vi "Training_Baseline_ICA.vi"(0 "Random_Repeat":i32=20, 1 "Random_num":i32=9, 3 "Experimentation_num":i32=2, 4 "rate":dbl=500.0 caption="Rate" format="%0.2f", 5 "Group Number":i32, 6 "Brain_data_source":dbl[](array[numeric]) caption="EEG_Raw_Data" format="%0.3f", 7 "samples per channel":i32=25, 9 "전체_Selected":i32[](array[numeric]), 10 "Selected":i32[](array[numeric]), 11 "Nontarget_Flash_Order":i32[][](array[numeric]), 12 "Target_Flash_Order":i64[](array[numeric]), 13 "W":dbl[][](array[numeric])) -> (14 "Target":dbl[][](array[numeric]), 15 "Nontarget_ERP":dbl[](array[numeric]), 18 "NonTarget":dbl[][](array[numeric]), 19 "Target_ERP":dbl[](array[numeric]))   [LabVIEW 2014]
uses:
  <vilib>/Analysis/3filter.llb/Filter Passband Type.ctl
  <vilib>/Analysis/baseanly.llb/Mean (DBL).vi
  <vilib>/Analysis/3filter.llb/Butterworth Filter (DBL).vi
  <vilib>/Analysis/NI_AALBase.lvlib
  <vilib>/gmath/NI_Gmath.lvlib
  <vilib>/Utility/file.llb/Read From Spreadsheet File (DBL).vi
panel:
  in  "nontarget order":path=path "C:/Users/Administrator/Desktop/공공복지안전사업연구-노수진/파일럿20130902/전선미1_Training_Test/nontarget_order.xls"
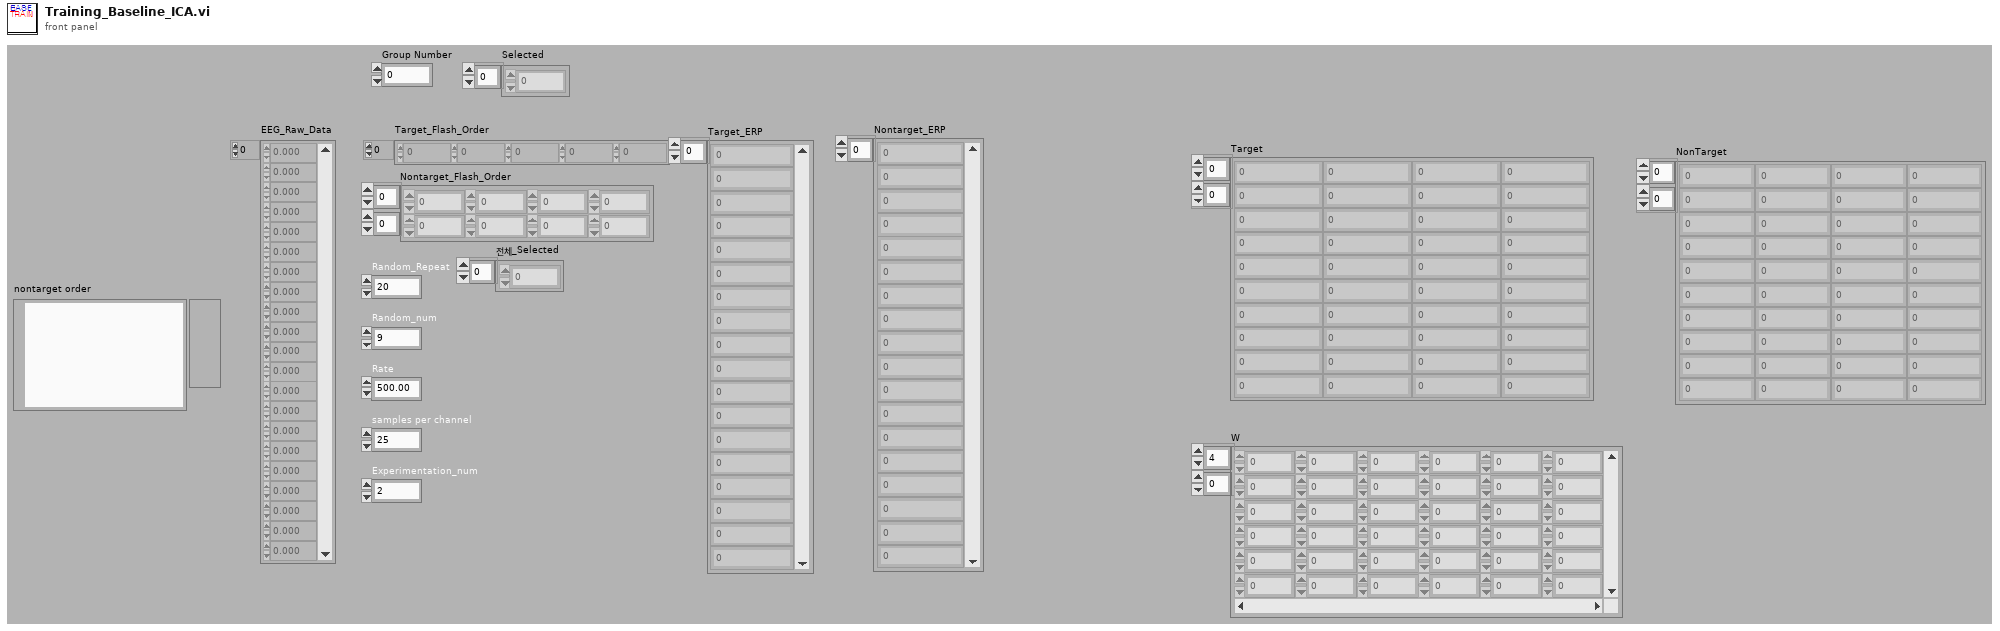
[diagram p1: front panel]
types:
  T1 = typedef "NI_AALBase.lvlib/Filter Passband Type.ctl" = enum32{"Lowpass", "Highpass", "Bandpass", "Bandstop"}
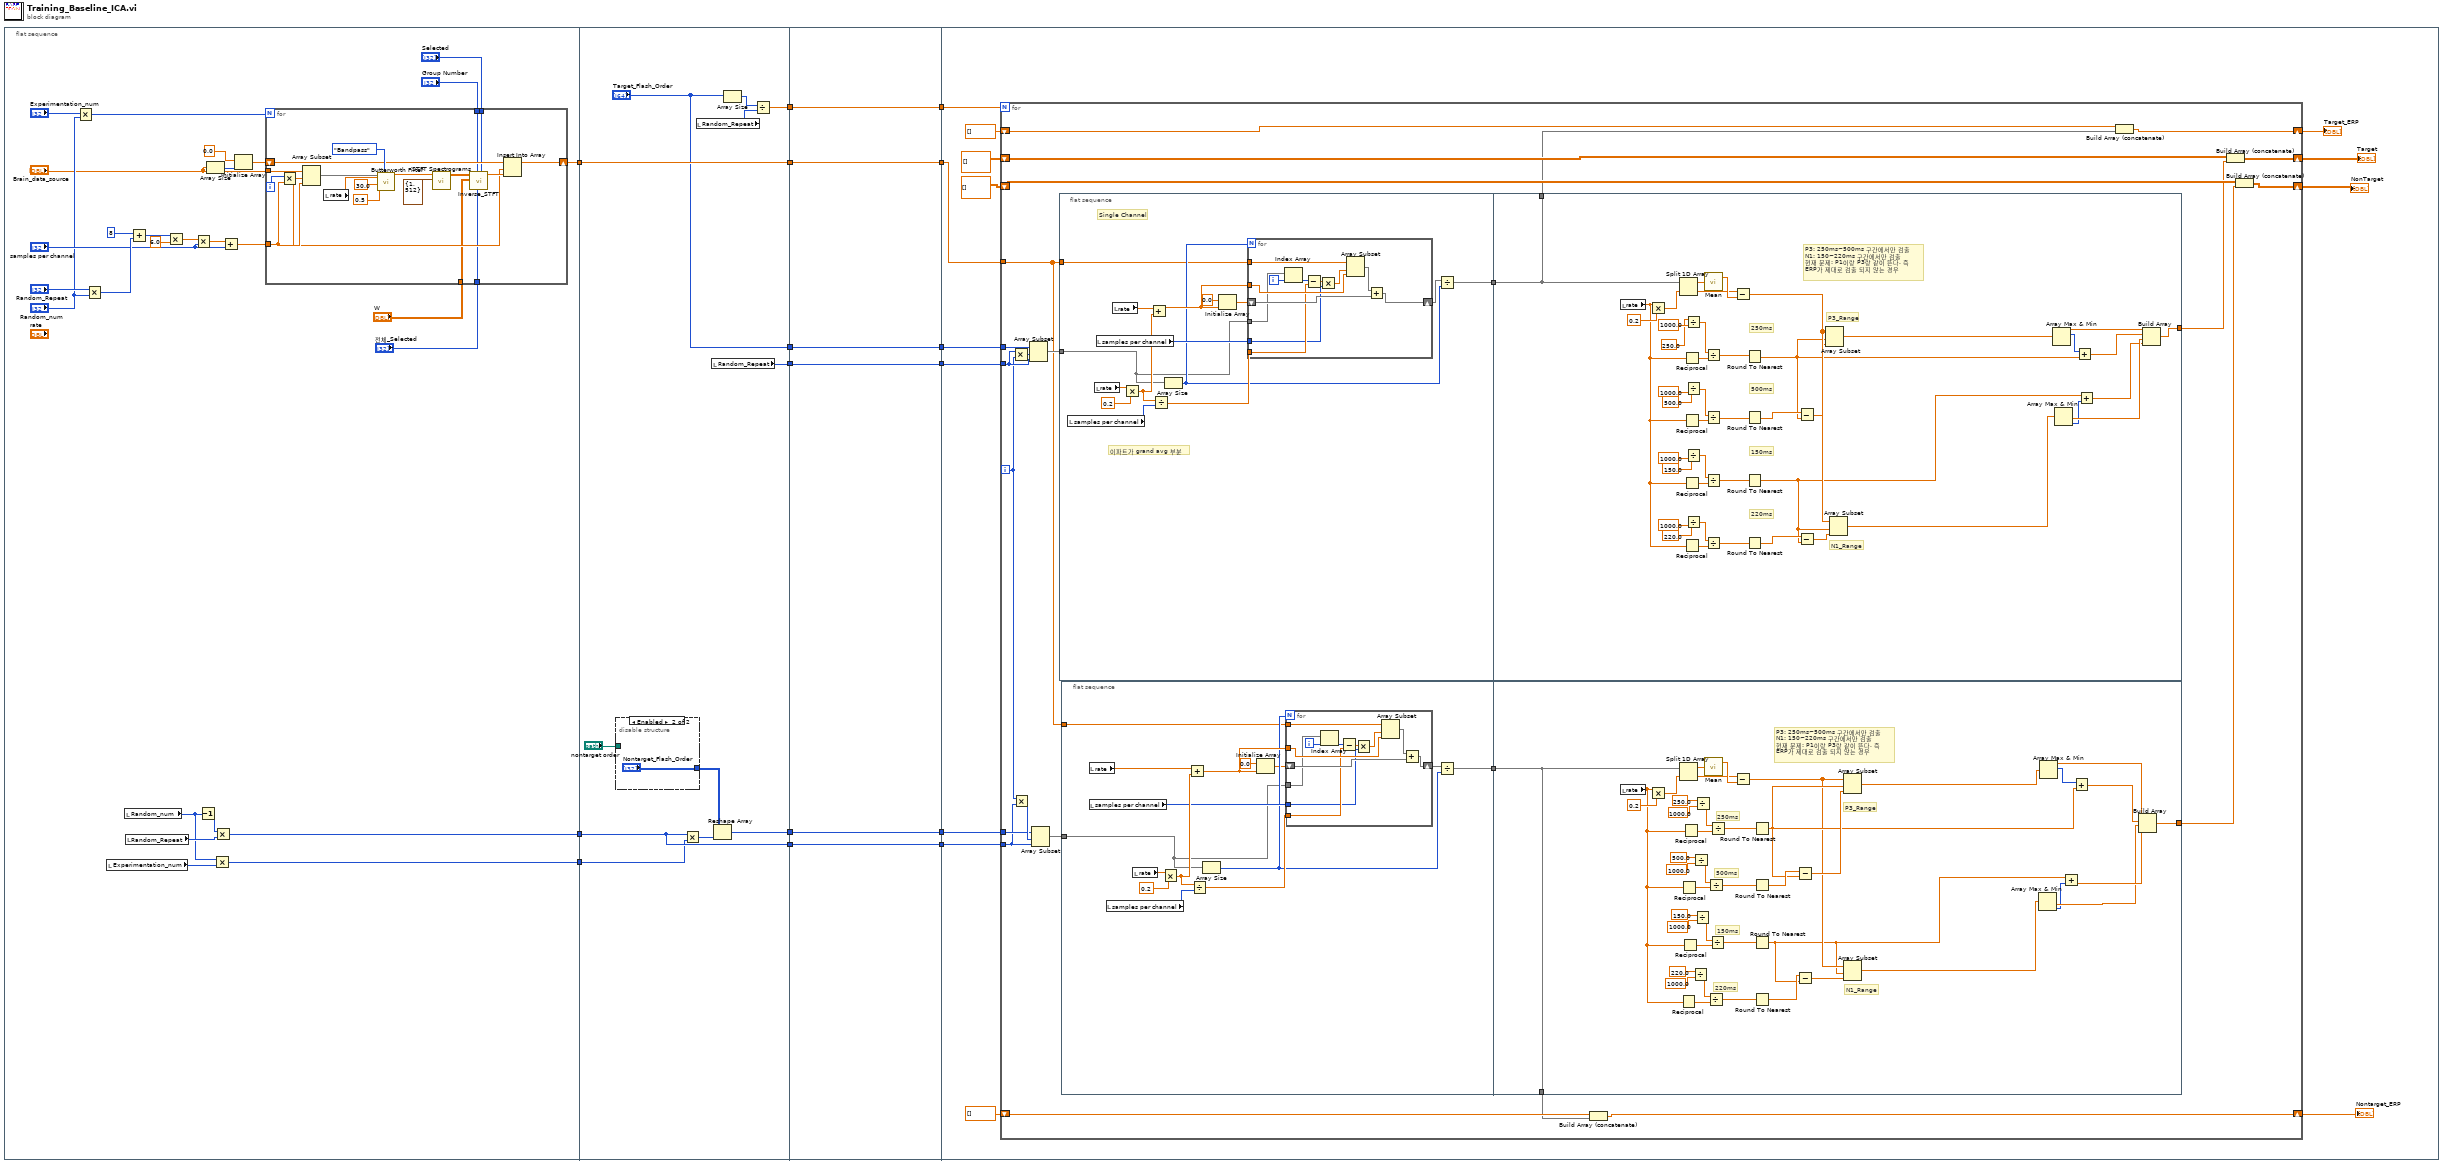
[diagram p0: block diagram]
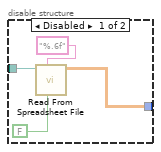
[diagram p2: hidden frame]
diagram:
  n1 = flat-sequence {
    tunnel: [w40] -> w3
    tunnel: [w42] -> w2
    tunnel: [w41] -> w1
    tunnel: w3 -> [w73]
    tunnel: [w73] -> w15
    tunnel: [w70] -> w13
    tunnel: ["Target_Flash_Order"] -> w11
    tunnel: [w69] -> w9
    tunnel: w2 -> [w66]
    tunnel: [w67] -> w7
    tunnel: [w66] -> w5
    tunnel: w1 -> [w65]
    tunnel: w15 -> [w79]
    tunnel: [w79] -> w14
    tunnel: w13 -> [w84]
    tunnel: [w84] -> w12
    tunnel: w11 -> [w83]
    tunnel: [w83] -> w10
    tunnel: w9 -> [w82]
    tunnel: [w82] -> w8
    tunnel: w7 -> [w81]
    tunnel: [w81] -> w6
    tunnel: w5 -> [w80]
    tunnel: [w80] -> w4
    tunnel: w14 -> [w98]
    tunnel: w12 -> [w89]
    tunnel: w10 -> [w97]
    tunnel: w8 -> [w96]
    tunnel: w6 -> [w95]
    tunnel: w4 -> [w94]
    frame #0 {
      n2 = Multiply(x="Experimentation_num", y="Random_num") -> (x*y=w25:i32)
      n3 = Multiply(x="Random_Repeat", y="Random_num") -> (x*y=w29:i32)
      n4 = local read "Experimentation_num"() -> (w37:i32)
      n5 = local read "Random_num"() -> (w36:i32)
      n6 = local read "Random_Repeat"() -> (w38:i32)
      n7 = Add(x=8, y=w29) -> (x+y=w34:i32)
      n8 = Multiply(x=w34, y=6.0) -> (x*y=w32:dbl)
      n9 = Multiply(x=w32, y="samples per channel") -> (x*y=w31:dbl)
      n10 = Decrement(x=w36) -> (x-1=w39:i32)
      n11 = Array Size(array="Brain_data_source") -> (size(s)=w22:i32)
      n12 = Multiply(x=w36, y=w37) -> (x*y=w41:i32)
      n13 = Multiply(x=w39, y=w38) -> (x*y=w42:i32)
      n14 = Add(x=w31, y="samples per channel") -> (x+y=w24:dbl)
      n15 = Initialize Array(0.0 ("element"), w22) -> (w23:dbl[])
      n16 = for {
        N: w25 -> [_]
        tunnel: "Brain_data_source" -> [w54]
        tunnel: w24 -> [w48]
        shift-right: [w51] -> w40
        shift-left: w23 -> [w49]
        tunnel: "Selected" -> [w46]
        tunnel: "Group Number" -> [w45]
        tunnel: "W" -> [w44]
        tunnel: "전체_Selected" -> [w43]
        i -> [w52]
        n17 = Multiply(x=w52, y=w48) -> (x*y=w47:dbl)
        n18 = Array Subset(array=w54, index=w47, length=w48) -> (w53:dbl[])
        n19 = local read "rate"() -> (w55:dbl)
        n20 = call-poly <vilib>:"Butterworth Filter.vi"("filter type"=Filter_Passband_Type."Bandpass", "low cutoff freq: fl"=0.5, "high cutoff freq: fh"=30.0, "sampling freq: fs"=w55, "X"=w53) -> ("Filtered X"=w61:dbl[])  [unwired: 3 in, 1 out]
        n21 = call <vilib>:"STFT Spectrograms.vi"("time-freq sampling info"=cluster{"time steps":i32, "frequency bins":i32} {"time steps"=1, "frequency bins"=512}, "X"=w61) -> ("STFT Spectrogram {X}"=w59:dbl[][])  [unwired: 8 in, 1 out]
        n22 = call "Inverse_STFT.vi"("Selected"=w46, "전체_Selected"=w43, "Group Number"=w45, "W"=w44, "STFT Spectrogram {X}"=w59) -> ("Inverse_STFT"=w50:dbl[])  [unwired: 6 in]
        n23 = Insert Into Array(array=w49, index=w47, new element=w50) -> (w51:dbl[])
      }
    }
    frame #1 {
      n24 = disable-structure shown="Enabled" {
        disable-tunnel: "nontarget order" -> [w77 _]
        disable-tunnel: [w75 "Nontarget_Flash_Order"] -> w63
        frame Disabled {
          n25 = call-poly <vilib>:"Read From Spreadsheet File.vi"("transpose (no:F)"=FALSE, "format (%.3f)"="%.6f", "file path (dialog if empty)"=w77) -> ("all rows"=w75:dbl[][])  [unwired: 4 in, 4 out]
        }
        frame Enabled {
        }
      }
      n26 = Multiply(x=w66, y=w65) -> (x*y=w68:i32)
      n27 = local read "Random_Repeat"() -> (w71:i32)
      n28 = local read "Random_Repeat"() -> (w69:i32)
      n29 = Reshape Array(w63, w68) -> (w67:i32[])
      n30 = Array Size(array="Target_Flash_Order") -> (size(s)=w72:i32)
      n31 = Divide(x=w72, y=w71) -> (x/y=w70:dbl)
    }
    frame #2 {
    }
    frame #3 {
      n32 = for {
        N: w89 -> [_]
        tunnel: w98 -> [w118]
        tunnel: w97 -> [w122]
        tunnel: w96 -> [w120]
        tunnel: w95 -> [w115]
        tunnel: w94 -> [w113]
        shift-right: [w111] -> w91
        shift-left: dbl[][] [] -> [w112]
        shift-right: [w110] -> w90
        shift-left: dbl[][] [] -> [w109]
        shift-right: [w105] -> w86
        shift-left: dbl[] [] -> [w103]
        shift-right: [w106] -> w85
        shift-left: dbl[] [] -> [w108]
        i -> [w116]
        n33 = Multiply(x=w120, y=w116) -> (x*y=w121:i32)
        n34 = Multiply(x=w116, y=w113) -> (x*y=w117:i32)
        n35 = Array Subset(array=w122, index=w121, length=w120) -> (w119:i64[])
        n36 = Array Subset(array=w115, index=w117, length=w113) -> (w114:i32[])
        n37 = flat-sequence {
          tunnel: w118 -> [w194]
          tunnel: w119 -> [w198]
          tunnel: [w193] -> w102
          tunnel: [w258] -> w100
          tunnel: [w220] -> w104
          tunnel: w102 -> [w220]
          frame #0 {
            # "Single Channel"
            # "이파트가 grand avg 부분"
            n38 = local read "samples per channel"() -> (w201:i32)
            n39 = local read "rate"() -> (w203:dbl)
            n40 = local read "samples per channel"() -> (w200:i32)
            n41 = local read "rate"() -> (w205:dbl)
            n42 = Multiply(x=w203, y=0.2) -> (x*y=w207:dbl)
            n43 = Add(x=w205, y=w207) -> (x+y=w206:dbl)
            n44 = Divide(x=w207, y=w201) -> (x/y=w204:dbl)
            n45 = Array Size(array=w198) -> (size(s)=w199:i32)
            n46 = Initialize Array(0.0 ("element"), w206) -> (w197:dbl[])
            n47 = for {
              N: w199 -> [_]
              shift-right: [w217] -> w195
              shift-left: w197 -> [w218]
              tunnel: w206 -> [w216]
              tunnel: w198 -> [w214]
              tunnel: w204 -> [w212]
              tunnel: w200 -> [w210]
              tunnel: w194 -> [w209]
              i -> [w215]
              n48 = Index Array(array=w214, index=w215) -> (element=w213:i64)
              n49 = Subtract(x=w213, y=w212) -> (x-y=w211:dbl)
              n50 = Multiply(x=w211, y=w210) -> (x*y=w219:dbl)
              n51 = Array Subset(array=w209, index=w219, length=w216) -> (w208:dbl[])
              n52 = Add(x=w208, y=w218) -> (x+y=w217:dbl[])
            }
            n53 = Divide(x=w195, y=w199) -> (x/y=w193:dbl[])
          }
          frame #1 {
            # "N1_Range"
            # "P3_Range"
            # "220ms"
            # "150ms"
            # "500ms"
            # "250ms"
            # "P3: 250ms~500ms 구간에서만 검출\nN1: 150~220ms 구간에서만 검출\n현재 문제: P1이랑 P3랑 같이 뜬다. 즉\nERP가 제대로 검출 되지 않는 경우"
            n54 = local read "rate"() -> (w250:dbl)
            n55 = Multiply(x=w250, y=0.2) -> (x*y=w256:dbl)
            n56 = Split 1D Array(array=w220, index=w256) -> (first subarray=w255:dbl[], second subarray=w251:dbl[])
            n57 = Reciprocal(x=w250) -> (1/x=w249:dbl)
            n58 = Reciprocal(x=w250) -> (1/x=w248:dbl)
            n59 = Reciprocal(x=w250) -> (1/x=w247:dbl)
            n60 = Reciprocal(x=w250) -> (1/x=w246:dbl)
            n61 = Divide(x=250.0, y=1000.0) -> (x/y=w245:dbl)
            n62 = Divide(x=500.0, y=1000.0) -> (x/y=w244:dbl)
            n63 = Divide(x=150.0, y=1000.0) -> (x/y=w243:dbl)
            n64 = Divide(x=220.0, y=1000.0) -> (x/y=w242:dbl)
            n65 = call-poly <vilib>:"Mean.vi"("X"=w255) -> ("mean"=w254:dbl)  [unwired: 1 out]
            n66 = Divide(x=w245, y=w249) -> (x/y=w233:dbl)
            n67 = Divide(x=w244, y=w248) -> (x/y=w232:dbl)
            n68 = Divide(x=w243, y=w247) -> (x/y=w231:dbl)
            n69 = Divide(x=w242, y=w246) -> (x/y=w230:dbl)
            n70 = Subtract(x=w251, y=w254) -> (x-y=w227:dbl[])
            n71 = Round To Nearest(number=w233) -> (nearest integer value=w226:dbl)
            n72 = Round To Nearest(number=w232) -> (nearest integer value=w229:dbl)
            n73 = Round To Nearest(number=w231) -> (nearest integer value=w224:dbl)
            n74 = Round To Nearest(number=w230) -> (nearest integer value=w228:dbl)
            n75 = Subtract(x=w229, y=w226) -> (x-y=w225:dbl)
            n76 = Subtract(x=w228, y=w224) -> (x-y=w223:dbl)
            n77 = Array Subset(array=w227, index=w226, length=w225) -> (w222:dbl[])
            n78 = Array Subset(array=w227, index=w224, length=w223) -> (w221:dbl[])
            n79 = Array Max & Min(array=w222) -> (max value=w262:dbl, max index (indices)=w253:i32)  [unwired: 2 out]
            n80 = Array Max & Min(array=w221) -> (min value=w260:dbl, min index (indices)=w252:i32)  [unwired: 2 out]
            n81 = Add(x=w253, y=w226) -> (x+y=w261:dbl)
            n82 = Add(x=w224, y=w252) -> (x+y=w259:dbl)
            n83 = Build Array(w262, w261, w260, w259) -> (w258:dbl[])
          }
        }
        n84 = flat-sequence {
          tunnel: w118 -> [w124]
          tunnel: w114 -> [w128]
          tunnel: [w123] -> w101
          tunnel: [w188] -> w99
          tunnel: [w150] -> w107
          tunnel: w101 -> [w150]
          frame #0 {
            n85 = local read "rate"() -> (w135:dbl)
            n86 = local read "samples per channel"() -> (w130:i32)
            n87 = local read "samples per channel"() -> (w131:i32)
            n88 = local read "rate"() -> (w133:dbl)
            n89 = Multiply(x=w133, y=0.2) -> (x*y=w137:dbl)
            n90 = Add(x=w135, y=w137) -> (x+y=w136:dbl)
            n91 = Divide(x=w137, y=w131) -> (x/y=w134:dbl)
            n92 = Array Size(array=w128) -> (size(s)=w129:i32)
            n93 = Initialize Array(0.0 ("element"), w136) -> (w127:dbl[])
            n94 = for {
              N: w129 -> [_]
              shift-right: [w147] -> w125
              shift-left: w127 -> [w148]
              tunnel: w136 -> [w146]
              tunnel: w128 -> [w144]
              tunnel: w134 -> [w142]
              tunnel: w130 -> [w140]
              tunnel: w124 -> [w139]
              i -> [w145]
              n95 = Index Array(array=w144, index=w145) -> (element=w143:i32)
              n96 = Subtract(x=w143, y=w142) -> (x-y=w141:dbl)
              n97 = Multiply(x=w141, y=w140) -> (x*y=w149:dbl)
              n98 = Array Subset(array=w139, index=w149, length=w146) -> (w138:dbl[])
              n99 = Add(x=w138, y=w148) -> (x+y=w147:dbl[])
            }
            n100 = Divide(x=w125, y=w129) -> (x/y=w123:dbl[])
          }
          frame #1 {
            # "N1_Range"
            # "P3_Range"
            # "220ms"
            # "150ms"
            # "500ms"
            # "250ms"
            # "P3: 250ms~500ms 구간에서만 검출\nN1: 150~220ms 구간에서만 검출\n현재 문제: P1이랑 P3랑 같이 뜬다. 즉\nERP가 제대로 검출 되지 않는 경우"
            n101 = local read "rate"() -> (w164:dbl)
            n102 = Multiply(x=w164, y=0.2) -> (x*y=w186:dbl)
            n103 = Split 1D Array(array=w150, index=w186) -> (first subarray=w185:dbl[], second subarray=w183:dbl[])
            n104 = Reciprocal(x=w164) -> (1/x=w168:dbl)
            n105 = Reciprocal(x=w164) -> (1/x=w176:dbl)
            n106 = Reciprocal(x=w164) -> (1/x=w172:dbl)
            n107 = Reciprocal(x=w164) -> (1/x=w180:dbl)
            n108 = Divide(x=220.0, y=1000.0) -> (x/y=w165:dbl)
            n109 = Divide(x=500.0, y=1000.0) -> (x/y=w173:dbl)
            n110 = Divide(x=150.0, y=1000.0) -> (x/y=w169:dbl)
            n111 = Divide(x=250.0, y=1000.0) -> (x/y=w177:dbl)
            n112 = call-poly <vilib>:"Mean.vi"("X"=w185) -> ("mean"=w184:dbl)  [unwired: 1 out]
            n113 = Divide(x=w165, y=w168) -> (x/y=w160:dbl)
            n114 = Divide(x=w173, y=w176) -> (x/y=w162:dbl)
            n115 = Divide(x=w169, y=w172) -> (x/y=w161:dbl)
            n116 = Divide(x=w177, y=w180) -> (x/y=w163:dbl)
            n117 = Subtract(x=w183, y=w184) -> (x-y=w153:dbl[])
            n118 = Round To Nearest(number=w163) -> (nearest integer value=w157:dbl)
            n119 = Round To Nearest(number=w162) -> (nearest integer value=w159:dbl)
            n120 = Round To Nearest(number=w161) -> (nearest integer value=w151:dbl)
            n121 = Round To Nearest(number=w160) -> (nearest integer value=w154:dbl)
            n122 = Subtract(x=w159, y=w157) -> (x-y=w158:dbl)
            n123 = Subtract(x=w154, y=w151) -> (x-y=w155:dbl)
            n124 = Array Subset(array=w153, index=w157, length=w158) -> (w156:dbl[])
            n125 = Array Subset(array=w153, index=w151, length=w155) -> (w152:dbl[])
            n126 = Array Max & Min(array=w152) -> (min value=w189:dbl, min index (indices)=w182:i32)  [unwired: 2 out]
            n127 = Array Max & Min(array=w156) -> (max value=w192:dbl, max index (indices)=w181:i32)  [unwired: 2 out]
            n128 = Add(x=w151, y=w182) -> (x+y=w190:dbl)
            n129 = Add(x=w181, y=w157) -> (x+y=w191:dbl)
            n130 = Build Array(w192, w191, w189, w190) -> (w188:dbl[])
          }
        }
        n131 = Build Array (concatenate)(w108, w107) -> (w106:dbl[])
        n132 = Build Array (concatenate)(w103, w104) -> (w105:dbl[])
        n133 = Build Array (concatenate)(w112, w100) -> (w111:dbl[][])
        n134 = Build Array (concatenate)(w109, w99) -> (w110:dbl[][])
      }
      "Target" <- w91
      "NonTarget" <- w90
      "Target_ERP" <- w86
      "Nontarget_ERP" <- w85
    }
  }
